vi "Linux.vi"(8 "error in (no error)":errorcluster, 10 "Font in":string, 11 "Font":refnum<vi>) -> (0 "error out":errorcluster, 2 "Font out":string)   [LabVIEW 2021]
uses:
  <vilib>/LabVIEW Icon API/lv_icon/lv_icon.lvlib
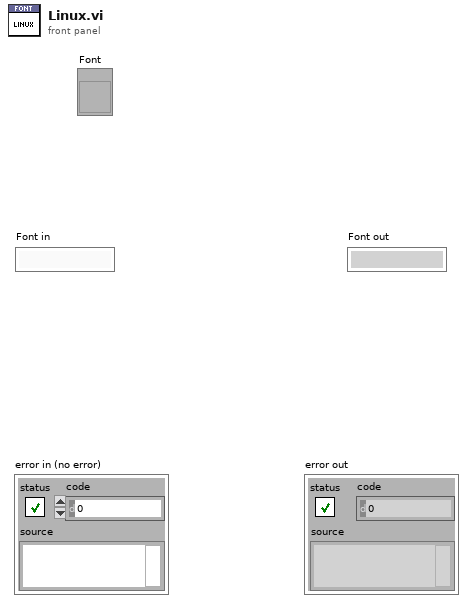
[diagram p1: front panel]
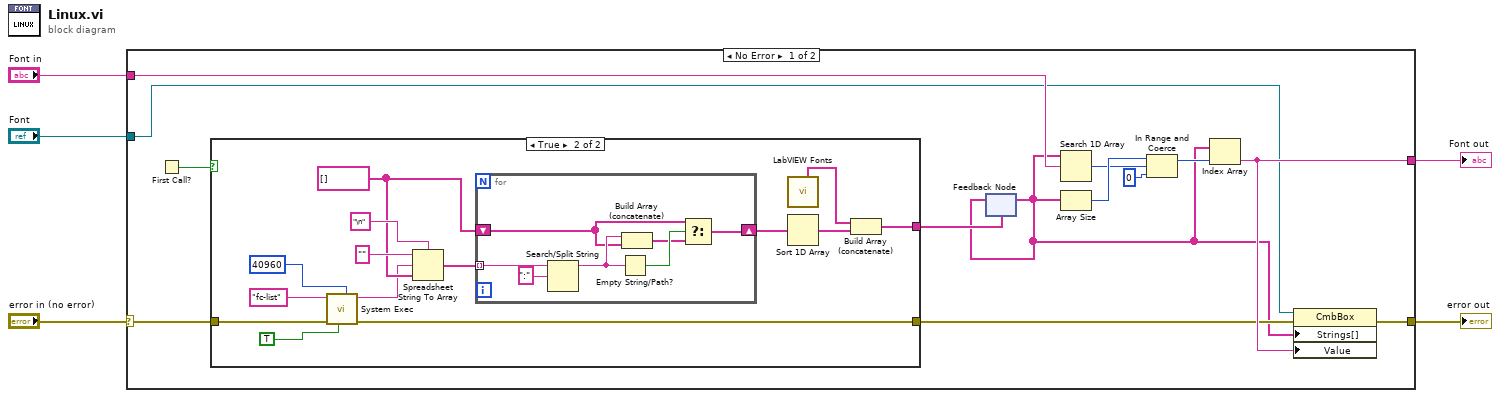
[diagram p0: block diagram]
diagram:
  n1 = case shown="No Error" "error in (no error)" {
    selector: "error in (no error)" -> [w18 w42]
    tunnel: [w17 w42] -> w4
    tunnel: "Font in" -> [w12 w41]
    tunnel: [w11 w41] -> w2
    tunnel: "Font" -> [w10 _]
    frame No Error {
      n2 = First Call?() -> (First Call?: T/F=w6:bool)
      n3 = case shown="True" w6 {
        tunnel: w18 -> [w19 w25]
        tunnel: [w19 w21] -> w9
        tunnel: [_ w20] -> w8
        frame False {
        }
        frame True {
          w27 = string[] []
          n4 = call <vilib>:"System Exec.vi"("expected output size  (4096)"=u32 40960, "run minimized? (F)"=TRUE, "error in (no error)"=w25, "command line"="fc-list") -> ("error out"=w21:errorcluster, "standard output"=w24:string)  [unwired: 3 in, 3 out]
          n5 = Spreadsheet String To Array(delimiter (Tab)="\n", format string="", spreadsheet string=w24, array type (2D Dbl)=w27) -> (array=w28:string[])
          n6 = for {
            tunnel: w28 -> [w40] mode=indexing
            shift-right: [w34] -> w26
            shift-left: w27 -> [w36]
            n7 = Search/Split String(string=w40, search string/char (-)=":") -> (substring before match=w37:string)  [unwired: 3 out]
            n8 = Empty String/Path?(string/path=w37) -> (empty?=w38:bool)
            n9 = Build Array (concatenate)(w37, w36) -> (w35:string[])
            n10 = Select(t=w36, s=w38, f=w35) -> (s? t:f=w34:string[])
          }
          n11 = call <vilib>:"LabVIEW Fonts.vi"() -> ("Additional Fonts"=w22:string[])  [unwired: 1 in, 10 out]
          n12 = Sort 1D Array(array=w26) -> (sorted array=w23:string[])
          n13 = Build Array (concatenate)(w22, w23) -> (w20:string[])
        }
      }
      n14 = feedback #1(w8) -> (w7:string[])
      n15 = feedback-in #1(w7) -> ()
      n16 = Search 1D Array(1D array=w7, element=w12) -> (index of element=w13:i32)  [unwired: 1 out]
      n17 = Array Size(array=w7) -> (size(s)=w16:i32)
      n18 = In Range and Coerce(upper limit=w16, x=w13, lower limit=0 ("x")) -> (coerced(x)=w15:i32)  [unwired: 1 out]
      n19 = Index Array(array=w7, index=w15) -> (element=w11:string)
      n20 = property class="CmbBox"(reference=w10, error in=w9, "Strings[]"=w7, "Value"=w11) -> (error out=w17:errorcluster)  [unwired: 1 out]
    }
    frame Error {
    }
  }
  "error out" <- w4
  "Font out" <- w2
